vi "Prepare Results.vi"(8 "error in (no error)":errorcluster, 9 "Execution Time":dbl, 11 "LUnit Test Case In":refnum<class "LUnit Inheriting Test Case.lvclass">) -> (0 "error out":errorcluster, 2 "Results":T1[](array[typedef]), 3 "LUnit Test Case Out":refnum<class "LUnit Inheriting Test Case.lvclass">)   [LabVIEW 2020]
uses:
  LUnit Inheriting Test Case.lvclass/LUnit Inheriting Test Case.ctl
  Core/Result/Type.ctl
  Core/Result/Result.lvlib
  Core/Result/Status.ctl
  Core/Result/Result.ctl
  LUnit Inheriting Test Case.lvclass
  C:/git/astemes-lunit/source/API/LUnit Test Case/LUnit Test Case.lvclass
  C:/git/astemes-lunit/source/Core/Runnable/Runnable.lvclass
  C:/git/astemes-lunit/source/API/LUnit Inheriting Test Case/LUnit Test Case/LUnit Inheriting Test Case.lvclass
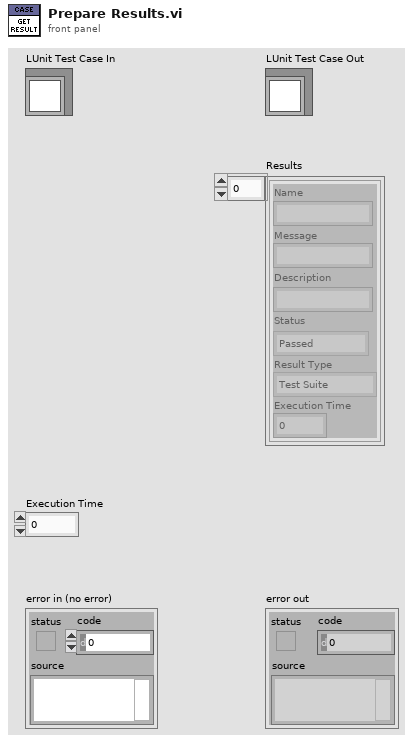
[diagram p1: front panel]
types:
  T1 = typedef "Result.lvlib/Result.ctl" = cluster{"Name":string, "Message":string, "Description":string, "Status":T2, "Result Type":T3, "Execution Time":dbl}
  T2 = typedef "Result.lvlib/Status.ctl" = enum16{"", "Passed", "Failed", "Error", "Skipped", "Setup Error", "Broken", "Teardown Error"}
  T3 = typedef "Result.lvlib/Type.ctl" = enum16{"Test Case", "Test Suite", "Test Run", "Pass", "Fail", "Skip", "Pass if", "Fail if", "Pass if Error", "Fail if Error", "Pass if Equal", "Fail if Equal"}
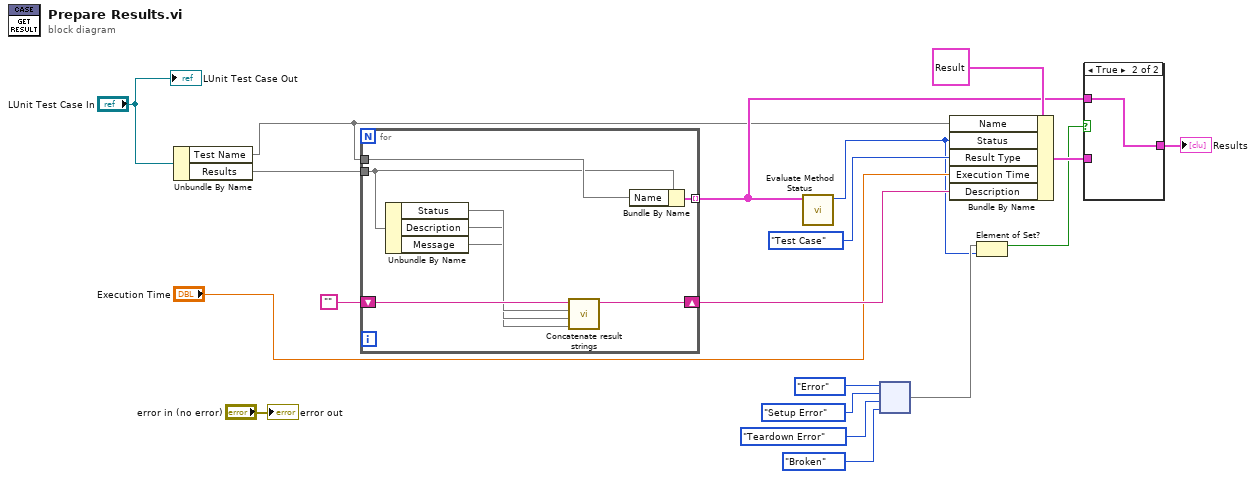
[diagram p0: block diagram]
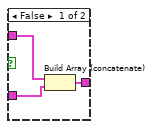
[diagram p2: hidden frame]
diagram:
  n1 = Unbundle By Name("LUnit Test Case In") -> ("Test Name"=w1, "Results"=w18)
  n2 = for {
    tunnel: w18 -> [w24]
    tunnel: w1 -> [w27]
    tunnel: [w26] -> w15 mode=indexing
    shift-right: [w20] -> w10
    shift-left: "" ("Input String") -> [w25]
    n3 = Unbundle By Name(w24) -> ("Status"=w23, "Description"=w22, "Message"=w21)
    n4 = call "Concatenate result strings.vi"("Message"=w21, "Description"=w22, "Status"=w23, "Input String"=w25) -> ("Output String"=w20:string)  [unwired: 7 in]
    n5 = Bundle By Name(cluster=w24, "Name"=w27) -> (w26:cluster{})
  }
  n6 = call "Evaluate Method Status.vi"("Results"=w15) -> ("Status"=w3:T2)  [unwired: 10 in]
  n7 = node(Status."Error" ("Status"), Status."Setup Error" ("Status"), Status."Teardown Error" ("Status"), Status."Broken" ("Status")) -> (w4:set{T2})
  n8 = Bundle By Name(cluster=T1 {"Name"="", "Message"="", "Description"="", "Status"=enum."Passed", "Result Type"=enum."Test Case", "Execution Time"=0.0} ("Results"), "Name"=w1, "Status"=w3, "Result Type"=Type."Test Case", "Execution Time"="Execution Time", "Description"=w10) -> (w13:T1)
  n9 = Element of Set?(10:w3, 11:w4) -> (3:w2:bool)
  n10 = case shown="True" w2 {
    tunnel: w15 -> [w30 w31]
    tunnel: [w29 w31] -> w14
    tunnel: w13 -> [w28 _]
    frame False {
      n11 = Build Array (concatenate)(w30, w28) -> (w29:T1[])
    }
    frame True {
    }
  }
  "Results" <- w14
  "error out" <- "error in (no error)"
  "LUnit Test Case Out" <- "LUnit Test Case In"
